vi "stringScalar.vi"(4 "String":string, 5 "msg in":string) -> (2 "msg out":string)   [LabVIEW 2013]
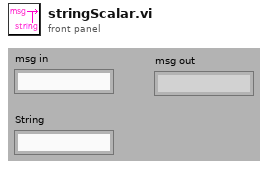
[diagram p1: front panel]
types:
  T1 = enum16{"big-endian, network order", "native, host order", "little-endian"}
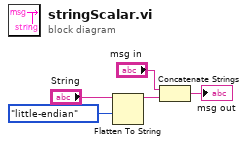
[diagram p0: block diagram]
diagram:
  n1 = Flatten To String(anything="String", byte order (0:big-endian, network order)=T1."little-endian") -> (data string=w4:string)  [unwired: 2 in, 2 out]
  n2 = Concatenate Strings("msg in", w4) -> (→"msg out":string)
